vi "all-signals-expressvi-to-TDMS-03-loop+time.vi"() -> ()   [LabVIEW 2018]
panel:
  in  "Dateipfad":path=path "C:/Users/lauri/OneDrive/Dokumente/Uni/HTW/Diplomarbeit/Versuchsstand neu/labview/messungen"
  in  "Stop Measurement (F)":bool caption="Messung stoppen, Counter schreiben (F)"
  in  "Clear Charts":bool
  in  "Messzeit in ms":u32=100 min=10 max=1000 step=10
  out "Bremsmoment":waveform(dbl)(graph)
  out "Strom, Spannung, elektrische Leistung":dynamicdata(graph)
  out "Counter/Messzeit":waveform(dbl)(graph)
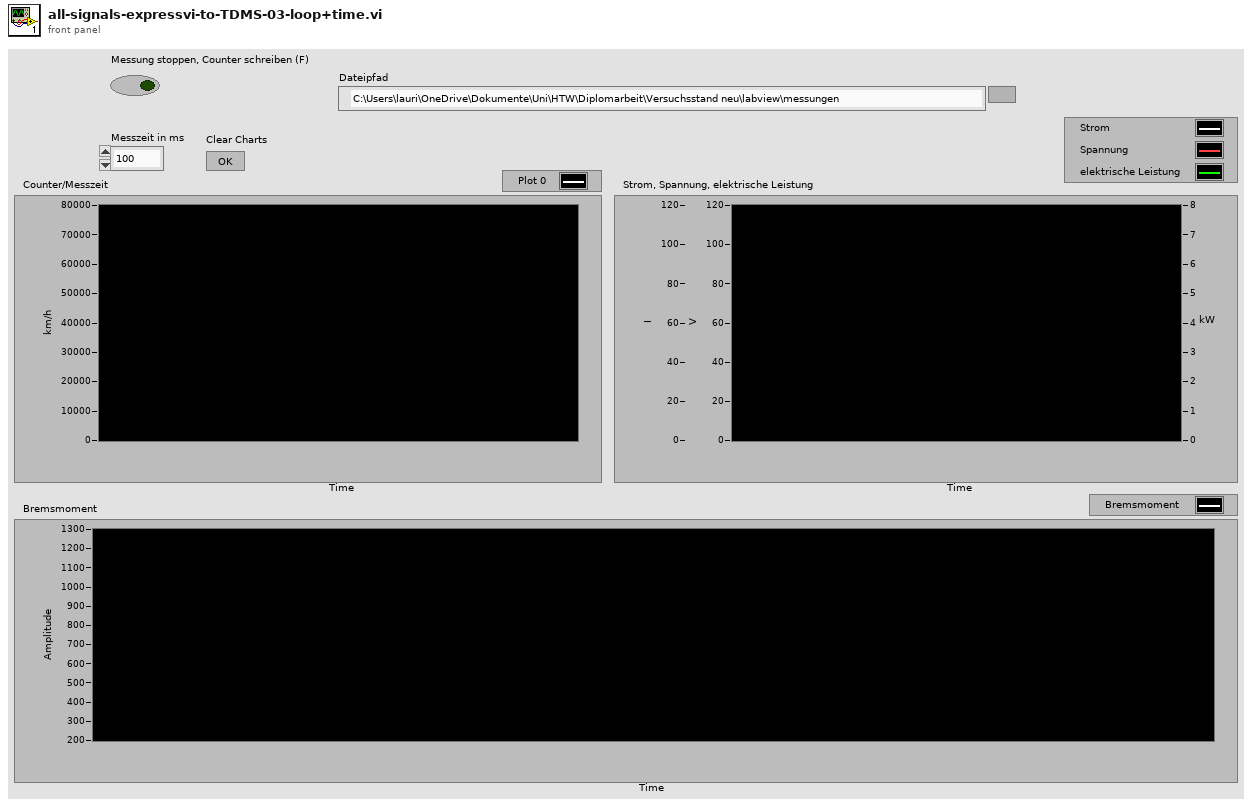
[diagram p1: front panel]
types:
  T1 = enum16{"open", "open or create", "create or replace", "create", "open (read-only)"}
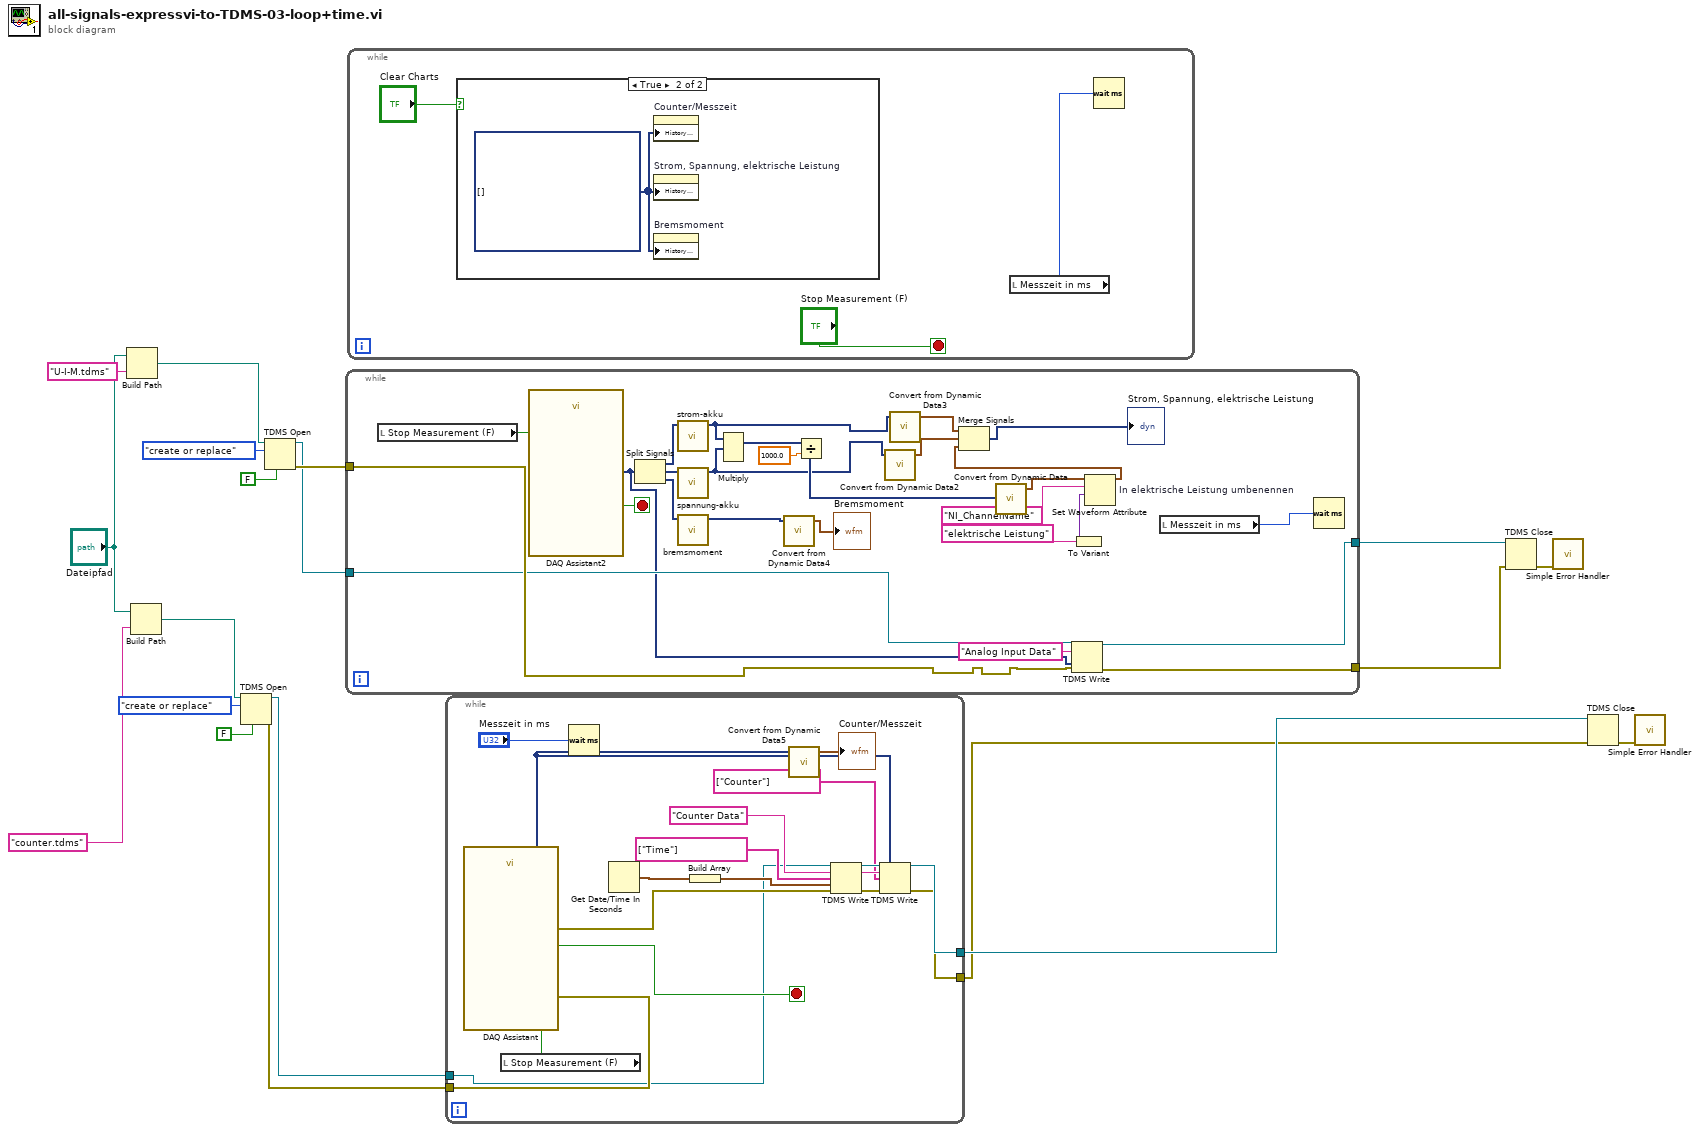
[diagram p0: block diagram]
diagram:
  n1 = Build Path(base path="Dateipfad", name or relative path="U-I-M.tdms") -> (appended path=w6:path)
  n2 = Build Path(base path="Dateipfad", name or relative path="counter.tdms" ("Dateiname")) -> (appended path=w9:path)
  n3 = TDMS Open(6:FALSE ("disable buffering? (T)"), 10:T1."create or replace" ("operation (0:open)"), 11:w9) -> (0:w19:errorcluster, 3:w14:refnum<k34>)  [unwired: 4 in]
  n4 = TDMS Open(6:FALSE ("disable buffering? (T)"), 10:T1."create or replace" ("operation (0:open)"), 11:w6) -> (0:w5:errorcluster, 3:w4:refnum<k34>)  [unwired: 4 in]
  n5 = while {
    tunnel: w5 -> [w23]
    tunnel: w4 -> [w22]
    tunnel: [w25] -> w2
    tunnel: [w24] -> w1
    stop <- w43 stop-if-true
    n6 = local read "Stop Measurement (F)"() -> (w40:bool)
    n7 = call "DAQ Assistant2"("stop (F)"=w40) -> ("data"=w21:dynamicdata, "stopped"=w43:bool)  [unwired: 15 in, 2 out]
    n8 = Split Signals(w21) -> (w46:dynamicdata, w45:dynamicdata, w44:dynamicdata)  [unwired: 3 in]
    n9 = call "strom-akku.vi"("Dynamic Data"=w46) -> ("Filtered Signal"=w31:dynamicdata)  [unwired: 10 in]
    n10 = call "spannung-akku.vi"("Dynamic Data in"=w45) -> ("Dynamic Data out"=w33:dynamicdata)  [unwired: 10 in]
    n11 = call "bremsmoment.vi"("Dynamic Data in"=w44) -> ("Dynamic Data out"=w27:dynamicdata)  [unwired: 10 in]
    n12 = Multiply(1:w33, 2:w31) -> (0:w41:dynamicdata)  [unwired: 1 in, 1 out]
    n13 = call "Convert from Dynamic Data4"("Dynamic Data Type"=w27) -> ("Waveform"=→"Bremsmoment":waveform(dbl))  [unwired: 3 in]
    n14 = Divide(x=w41, y=1000.0) -> (x/y=w39:dynamicdata)
    n15 = call "Convert from Dynamic Data2"("Dynamic Data Type"=w33) -> ("Waveform"=w32:waveform(dbl))  [unwired: 3 in]
    n16 = call "Convert from Dynamic Data3"("Dynamic Data Type"=w31) -> ("Waveform"=w30:waveform(dbl))  [unwired: 3 in]
    n17 = call "Convert from Dynamic Data"("Dynamic Data Type"=w39) -> ("Waveform"=w35:waveform(dbl))  [unwired: 3 in]
    n18 = TDMS Write(0:w22, 5:"Analog Input Data" ("group name in (Untitled)"), 9:w21, 11:w23) -> (4:w25:refnum<k34>, 15:w24:errorcluster)  [unwired: 2 in, 2 out]
    n19 = To Variant(anything="elektrische Leistung") -> (Variant=w38:variant)
    n20 = Set Waveform Attribute "In elektrische Leistung umbenennen"(5:w38, 6:"NI_ChannelName" ("name"), 7:w35) -> (3:w34:waveform(dbl))  [unwired: 1 in, 2 out]
    n21 = Merge Signals "Merge Signals"(w30, w32, w34) -> (→"Strom, Spannung, elektrische Leistung":dynamicdata)
    n22 = local read "Messzeit in ms"() -> (w28:u32)
    n23 = Wait (ms)(milliseconds to wait=w28) -> ()  [unwired: 1 out]
  }
  n24 = while {
    stop <- "Stop Measurement (F)" stop-if-true
    n25 = case shown="True" "Clear Charts" {
      frame False {
      }
      frame True {
        w50 = dynamicdata[] [] ("History Data")
        n26 = property on="Counter/Messzeit" class="WFChart (strict)"("History Data"=w50) -> ()  [unwired: 2 in, 2 out]
        n27 = property on="Strom, Spannung, elektrische Leistung" class="WFChart (strict)"("History Data"=w50) -> ()  [unwired: 2 in, 2 out]
        n28 = property on="Bremsmoment" class="WFChart (strict)"("History Data"=w50) -> ()  [unwired: 2 in, 2 out]
      }
    }
    n29 = local read "Messzeit in ms"() -> (w47:u32)
    n30 = Wait (ms)(milliseconds to wait=w47) -> ()  [unwired: 1 out]
  }
  n31 = while {
    tunnel: w19 -> [w66]
    tunnel: w14 -> [w53]
    tunnel: [w64] -> w13
    tunnel: [w63] -> w12
    stop <- w68 stop-if-true
    n32 = local read "Stop Measurement (F)"() -> (w67:bool)
    n33 = call "DAQ Assistant"("error in"=w66, "stop (F)"=w67) -> ("data"=w61:dynamicdata, "stopped"=w68:bool, "error out"=w60:errorcluster)  [unwired: 14 in, 1 out]
    n34 = Wait (ms)(milliseconds to wait="Messzeit in ms") -> ()  [unwired: 1 out]
    n35 = Get Date/Time In Seconds() -> (seconds since 1Jan1904=w55:timestamp)
    n36 = Build Array(w55) -> (w54:timestamp[])
    n37 = call "Convert from Dynamic Data5"("Dynamic Data Type"=w61) -> ("Waveform"=→"Counter/Messzeit":waveform(dbl))  [unwired: 3 in]
    n38 = TDMS Write(0:w53, 5:"Counter Data" ("group name in (Untitled)"), 7:string[] ["Time"] ("channel name(s) in (Untitled)"), 9:w54, 11:w60) -> (4:w52:refnum<k34>, 6:w57:string, 15:w59:errorcluster)  [unwired: 1 in, 1 out]
    n39 = TDMS Write(0:w52, 5:w57, 7:string[] ["Counter"] ("channel name(s) in (Untitled)"), 9:w61, 11:w59) -> (4:w64:refnum<k34>, 15:w63:errorcluster)  [unwired: 1 in, 2 out]
  }
  n40 = TDMS Close(8:w1, 11:w2) -> (0:w3:errorcluster)  [unwired: 1 out]
  n41 = call <vilib>:"Simple Error Handler.vi"("error in (no error)"=w3) -> ()  [unwired: 2 in, 7 out]
  n42 = TDMS Close(8:w12, 11:w13) -> (0:w15:errorcluster)  [unwired: 1 out]
  n43 = call <vilib>:"Simple Error Handler.vi"("error in (no error)"=w15) -> ()  [unwired: 2 in, 7 out]
